vi "日期时间组合数组-带索引顺序排列.vi"(8 "排序模式":enum16{"从小到大", "从大到小"}(ring), 11 "数组输入":i32[][](array[numeric])) -> (0 "索引映射":i32[](array[numeric]), 3 "排序后":i32[][](array[numeric]))   [LabVIEW 2013]
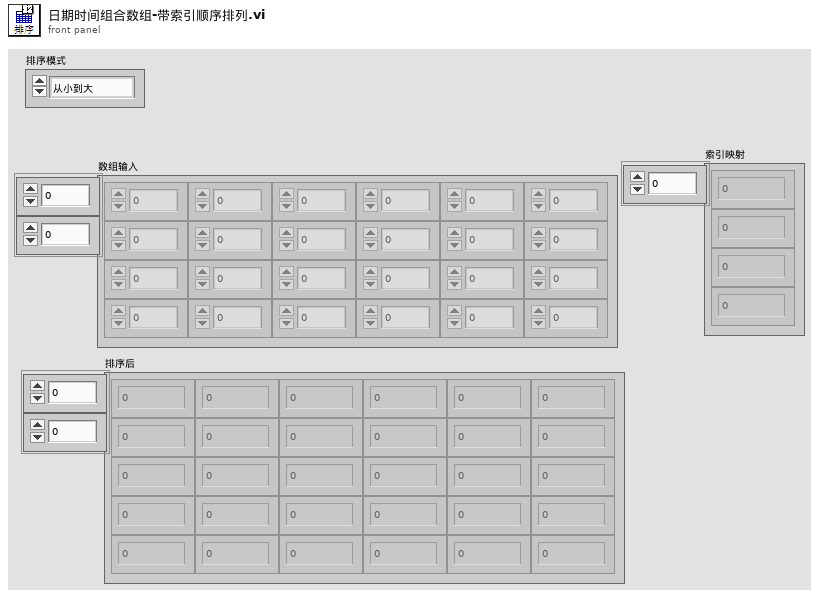
[diagram p1: front panel]
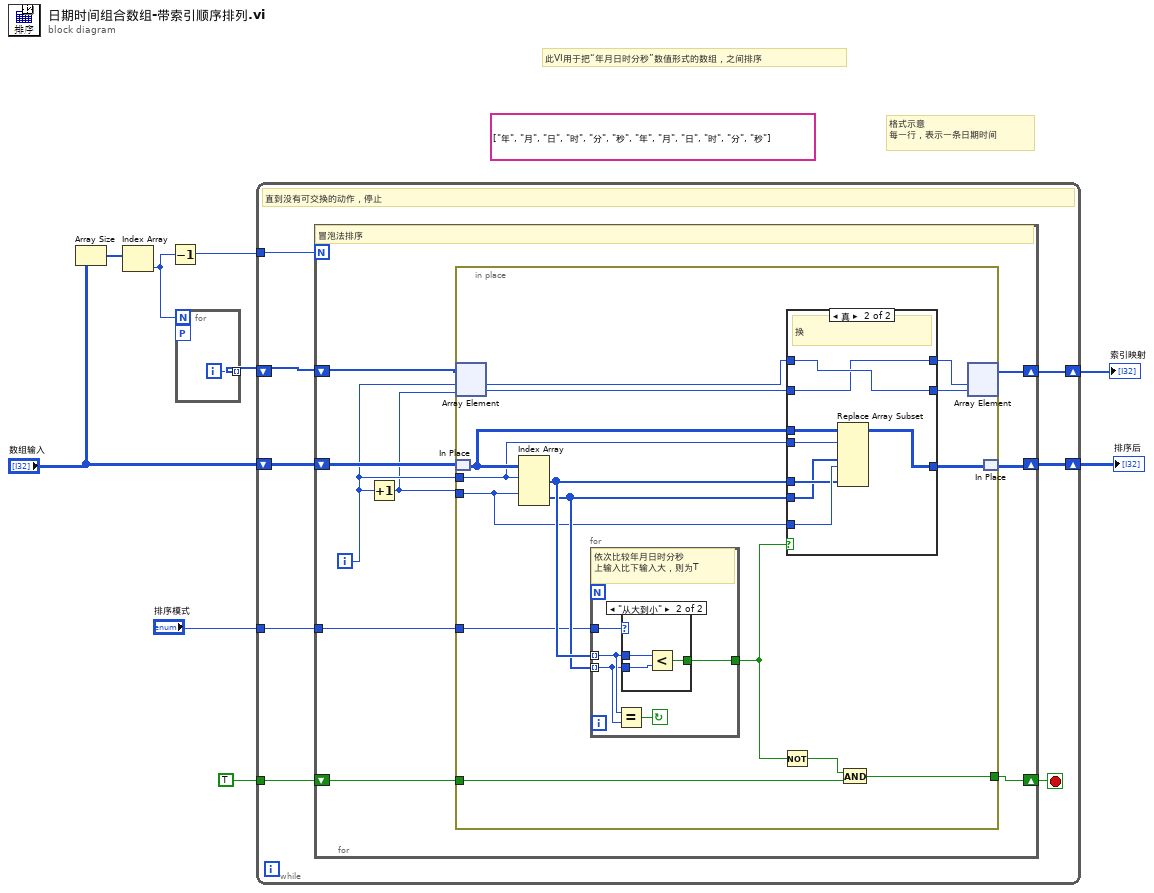
[diagram p0: block diagram]
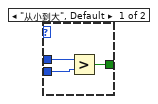
[diagram p2: hidden frame]
diagram:
  (unwired) string[][] [["年", "月", "日", "时", "分", "秒"], ["年", "月", "日", "时", "分", "秒"]]
  # "格式示意\n每一行，表示一条日期时间"
  # "此VI用于把“年月日时分秒”数值形式的数组，之间排序"
  n1 = Array Size(array="数组输入") -> (size(s)=w6:i32[])
  n2 = Index Array(array=w6) -> (element=w5:i32)  [unwired: 1 in]
  n3 = Decrement(x=w5) -> (x-1=w8:i32)
  n4 = for {
    N: w5 -> [_]
    workers-P: _ -> [_]
    tunnel: [w10] -> w9 mode=indexing
    i -> [w10]
  }
  n5 = while {
    tunnel: w8 -> [w16]
    shift-right: [w14] -> w7
    shift-left: "数组输入" -> [w18]
    shift-right: [w13] -> w2
    shift-left: w9 -> [w17]
    tunnel: "排序模式" -> [w12]
    tunnel: TRUE -> [w11]
    stop <- w15 stop-if-true
    # "直到没有可交换的动作，停止"
    n6 = for {
      N: w16 -> [_]
      shift-right: [w20] -> w14
      shift-left: w18 -> [w23]
      shift-right: [w26] -> w13
      shift-left: w17 -> [w27]
      shift-right: [w25] -> w15
      shift-left: w11 -> [w24]
      tunnel: w12 -> [w19]
      i -> [w22]
      # "冒泡法排序"
      n7 = Increment(x=w22) -> (x+1=w21:i32)
      n8 = in-place {
        in-place-border: [w36] -> w25
        in-place-border: w24 -> [w37]
        in-place-border: w22 -> [w31]
        in-place-border: w21 -> [w30]
        in-place-border: w19 -> [w29]
        n9 = in-place-array #1(w27, w22, w21) -> (w41:i32, w39:i32)
        n10 = in-place-match #2(w23) -> (w33:i32[][])
        n11 = Index Array(array=w33, index (row) #1=w31, index (row) #2=w30) -> (element #1=w35:i32[], element #2=w34:i32[])  [unwired: 2 in]
        n12 = for {
          tunnel: w35 -> [w46] mode=indexing
          tunnel: w34 -> [w45] mode=indexing
          tunnel: w29 -> [w44]
          tunnel: [w43] -> w28
          stop <- w47 continue-if-true
          # "依次比较年月日时分秒\n上输入比下输入大，则为T"
          n13 = Equal?(x=w46, y=w45) -> (x = y?=w47:bool)
          n14 = case shown="\"从大到小\"" w44 {
            tunnel: w46 -> [w50 w53]
            tunnel: w45 -> [w49 w52]
            tunnel: [w48 w51] -> w43
            frame "从小到大", Default {
              n15 = Greater?(x=w50, y=w49) -> (0:w48:bool)
            }
            frame "从大到小" {
              n16 = Less?(x=w53, y=w52) -> (x < y?=w51:bool)
            }
          }
        }
        n17 = Not(x=w28) -> (.not. x?=w38:bool)
        n18 = case shown="真" w28 {
          tunnel: w35 -> [_ w59]
          tunnel: w34 -> [_ w58]
          tunnel: [w55 w64] -> w42
          tunnel: w41 -> [w56 w64]
          tunnel: [w56 w63] -> w40
          tunnel: w39 -> [w55 w63]
          tunnel: w33 -> [w54 w62]
          tunnel: [w54 w57] -> w32
          tunnel: w31 -> [_ w61]
          tunnel: w30 -> [_ w60]
          frame False {
            # "不换"
          }
          frame True {
            # "换"
            n19 = Replace Array Subset(array=w62, new element #1=w58, index (row) #1=w61, new element #2=w59, index (row) #2=w60) -> (w57:i32[][])  [unwired: 2 in]
          }
        }
        n20 = And(x=w38, y=w37) -> (x .and. y?=w36:bool)
        n21 = in-place-array #1(w40, w42) -> (w26:i32[])  [unwired: 2 out]
        n22 = in-place-match #2(w32) -> (w20:i32[][])
      }
    }
  }
  "索引映射" <- w2
  "排序后" <- w7
